vi "serial_sweep_preset.vi"(11 "sweep_data":dbl[](array[numeric])) -> (1 "sweep_points":dbl, 2 "sweep_stop":dbl, 3 "sweep_start":dbl)   [LabVIEW 2025]
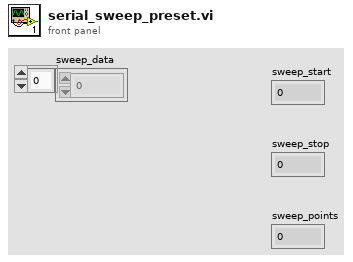
[diagram p1: front panel]
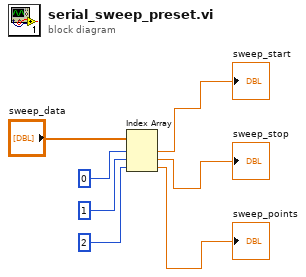
[diagram p0: block diagram]
diagram:
  n1 = Index Array(array="sweep_data", index #1=0 ("index"), index #2=1 ("index"), index #3=2 ("index")) -> (element #1=→"sweep_start":dbl, element #2=→"sweep_stop":dbl, element #3=→"sweep_points":dbl)
